vi "firstTimePeriodSolver.vi"(6 "initalVelocity":dbl, 9 "initalAccel":dbl, 10 "Array in":T1[](array[typedef]), 11 "Max profiles":T2) -> (3 "Array out":T1[](array[typedef]))   [LabVIEW 2014]
uses:
  TimeSegment.ctl
  Max profiles.ctl
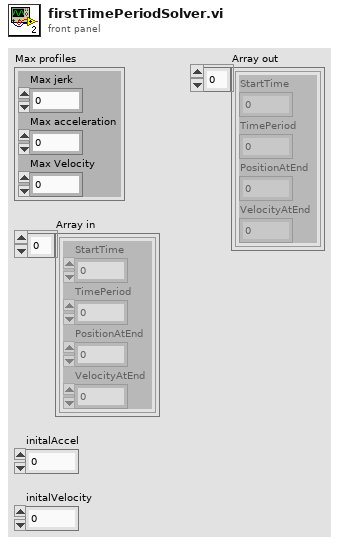
[diagram p1: front panel]
types:
  T1 = typedef "TimeSegment.ctl" = cluster{"StartTime":dbl, "TimePeriod":dbl, "PositionAtEnd":dbl, "VelocityAtEnd":dbl}
  T2 = typedef "Max profiles.ctl" = cluster{"Max jerk":dbl, "Max acceleration":dbl, "Max Velocity":dbl}
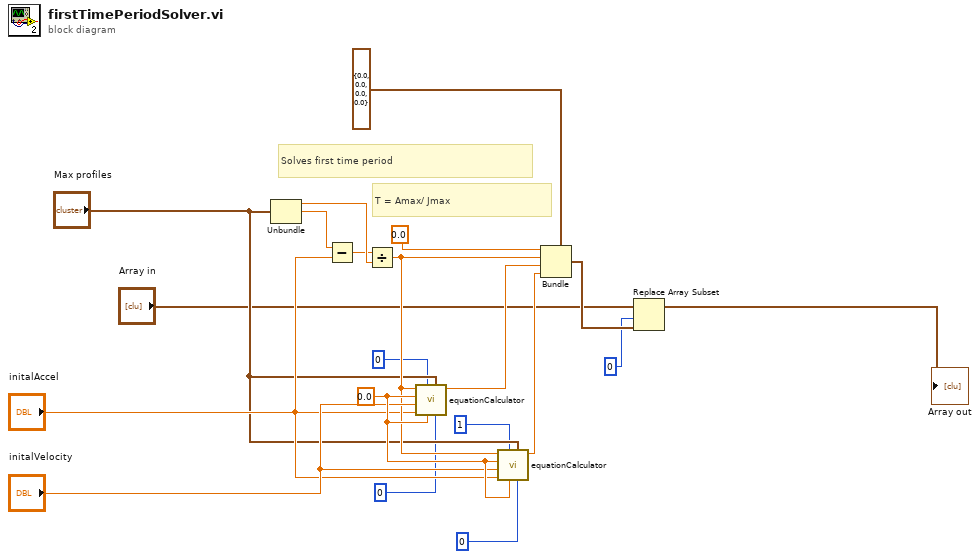
[diagram p0: block diagram]
diagram:
  w17 = 0.0 ("xInital")
  # "T = Amax/ Jmax"
  # "Solves first time period"
  n1 = Unbundle("Max profiles") -> ("Max jerk"=w5:dbl, "Max acceleration"=w3:dbl)  [unwired: 1 out]
  n2 = Subtract(x=w3, y="initalAccel") -> (x-y=w4:dbl)
  n3 = Divide(x=w4, y=w5) -> (x/y=w15:dbl)
  n4 = call "equationCalculator.vi"("Time Period"=i8 0, "Max profiles"="Max profiles", "startOfTimePeriod"=w17, "derivitave"=i8 0, "aInital (only needed for T0)"="initalAccel", "vInital"="initalVelocity", "xInital"=w17, "currentTime"=w15) -> ("output variable"=w19:dbl)  [unwired: 3 in]
  n5 = call "equationCalculator.vi"("Time Period"=i8 0, "Max profiles"="Max profiles", "startOfTimePeriod"=w17, "derivitave"=i8 1, "aInital (only needed for T0)"="initalAccel", "vInital"="initalVelocity", "xInital"=w17, "currentTime"=w15) -> ("output variable"=w18:dbl)  [unwired: 3 in]
  n6 = Bundle(cluster=T1 {"StartTime"=0.0, "TimePeriod"=0.0, "PositionAtEnd"=0.0, "VelocityAtEnd"=0.0} ("TimeSegment"), "StartTime"=0.0, "TimePeriod"=w15, "PositionAtEnd"=w19, "VelocityAtEnd"=w18) -> (w8:T1)
  n7 = Replace Array Subset(array="Array in", new element=w8, index=0) -> (→"Array out":T1[])
